vi "Actuators_N_Sensors.vi"() -> ()   [LabVIEW 2020]
panel:
  out "Auto Enabled":bool
  out "Enable Shooter Manipulation":bool
  out "Intake - Solenoid Manipulation":bool
  out "Climber Encoder":dbl
  out "Enable Shooter":bool
  out "Switch Hood":bool
  out "Shooter SetPoint Manipulation":dbl
  out "Kicker Wheel - Output Manipulation":dbl
  out "Omni - Output Manipulation":dbl
  out "Hood Encoder":dbl
  out "Turret Encoder":dbl
  out "Shooter SetPoint":dbl
  out "Hood SetPoint":dbl
  out "Turret SetPoint":dbl
  out "Aiming Enable":bool
  out "Hood - Output":dbl
  out "Turret - Output":dbl
  out "Shooter - Output":dbl
  out "DIO 5":bool
  out "DIO 1":bool
  out "DIO 4":bool
  out "DIO 3":bool
  out "DIO 0":bool
  out "DIO 2":bool
  out "ResetEncoderClimber":bool
  out "ResetEncoderDrivetrain":bool
  out "Compressor Off":bool
  out "ShooterRPM":dbl
  out "IR Conveyor":bool
  in  "Debug":dbl
  out "Intake - Output Manipulation":dbl
  out "Gyro - Yaw":dbl
  out "Gyro - Cont":dbl
  out "Climber - Output":dbl
  out "Climber - Solenoid":bool
  out "Intake - Solenoid":bool
  out "Kicker Wheel - Output":dbl
  out "Omni - Output":dbl
  out "Intake - Output":dbl
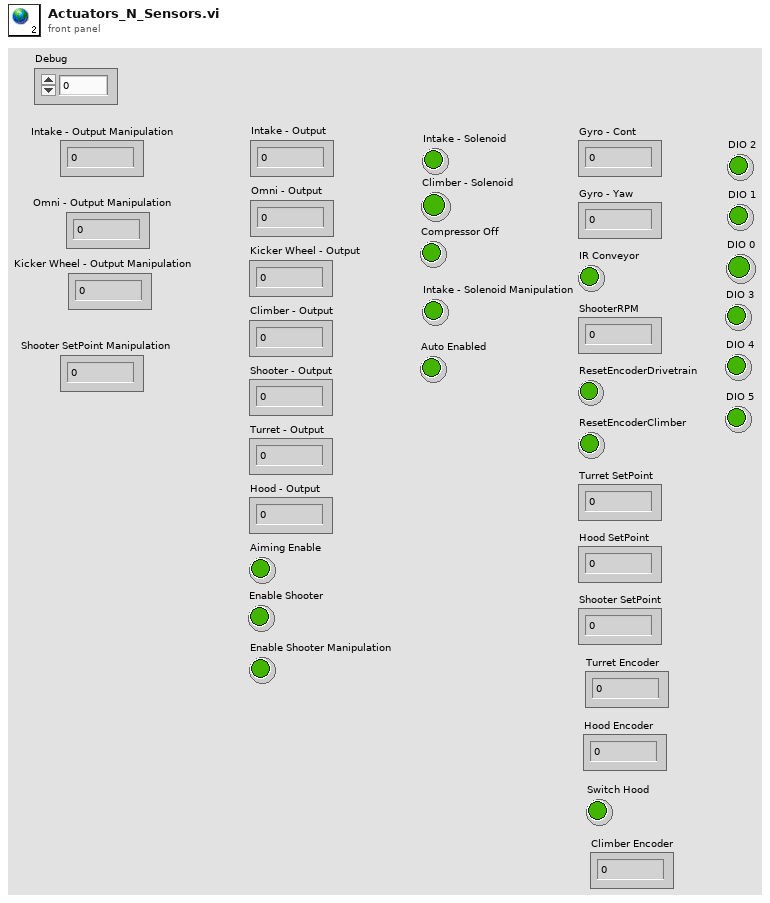
[diagram p1: front panel]
diagram:
